vi "init.vi"(8 "error in (no error)":errorcluster, 11 "ILC_TC in":refnum<class "ILC_TC.lvclass">) -> (0 "error out":errorcluster, 3 "ILC_TC out":refnum<class "ILC_TC.lvclass">)   [LabVIEW 2013, in "ILC_TC.lvclass"]
uses:
  ILC_TC.lvclass
  <userlib>/Common/ILC/Configuration/ILC Serial.ctl
  <userlib>/Common/SerialProtocols/Configuration/SerialConfig.ctl
  <userlib>/Common/SerialProtocols/Configuration/SerialProtocol.ctl
  <userlib>/Common/SerialProtocols/Configuration/ProtocolParameters.ctl
  <userlib>/Common/SerialProtocols/Configuration/SerialMessageParameters.ctl
  <userlib>/Common/ILC/Configuration/ILC ADC.ctl
  <userlib>/Common/ILC/Configuration/InputChannels.ctl
  <userlib>/Common/ILC/Configuration/ScanRate_Hz_MultichannelOptions.ctl
  <userlib>/Common/ILC/ILC/ILC.lvclass/ILC.ctl
  <userlib>/Common/ILC/ILC/ILC.lvclass
  <userlib>/Common/SerialProtocols/SerialProtocols.lvlib
  <userlib>/Common/ILC/Configuration/ILCConfiguration.lvlib
  ConfigurationThisComponent/ConfigurationThisComponent.lvclass
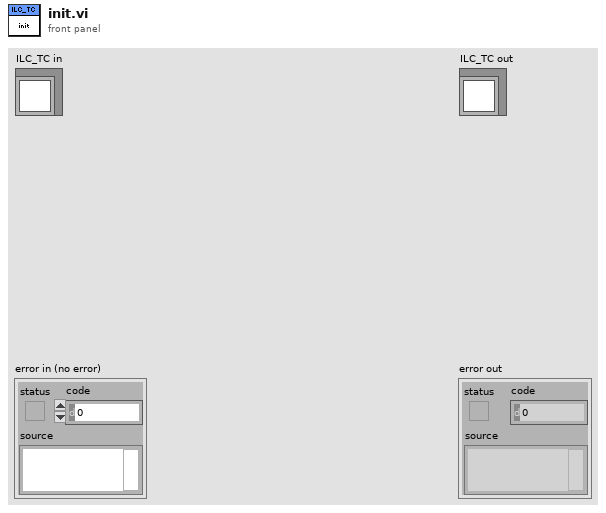
[diagram p1: front panel]
types:
  T1 = typedef "ILCCommon.lvlib/ILCConfiguration.lvlib/ILC ADC.ctl" = cluster{"Input Channels":T2, "Scan Rate (Hz) ":T3, "PGA Gain Coefficient":u8, "Reference Voltage Vref":dbl[unit], "Nominal Input Range in Counts":u32, "Preamplifier Gain":u8}
  T2 = typedef "ILCCommon.lvlib/ILCConfiguration.lvlib/InputChannels.ctl" = enum16{"Channel 0", "3 Channels", "5 Channels"}
  T3 = typedef "ILCCommon.lvlib/ILCConfiguration.lvlib/ScanRate_Hz_MultichannelOptions.ctl" = enum16{"50", "60", "100", "120", "200", "240", "300", "400", "480", "600", "1200", "2400", "4800"}
  T4 = typedef "ILCCommon.lvlib/ILCConfiguration.lvlib/ILC Serial.ctl" = cluster{"Serial":T5}
  T5 = typedef "SerialProtocols.lvlib/SerialConfig.ctl" = cluster{"Serial Protocol":T6, "Protocol Parameters":T7, "Serial Message Parameters":T8}
  T6 = typedef "SerialProtocols.lvlib/SerialProtocol.ctl" = enum16{"RS232", "RS485", "SerialSimulator"}
  T7 = typedef "SerialProtocols.lvlib/ProtocolParameters.ctl" = cluster{"VISA resource name":refnum<visa-resource-name>, "Baud Rate":u32, "Data Bits":u16, "Parity":enum16{"None", "Odd", "Even", "Mark", "Space"}, "Flow Control":u16, "Stop Bits":u16, "Timeout (ms)":u32}
  T8 = typedef "SerialProtocols.lvlib/SerialMessageParameters.ctl" = cluster{"Byte Count":u32, "Enable Termination Character":bool, "Termination Char":u8}
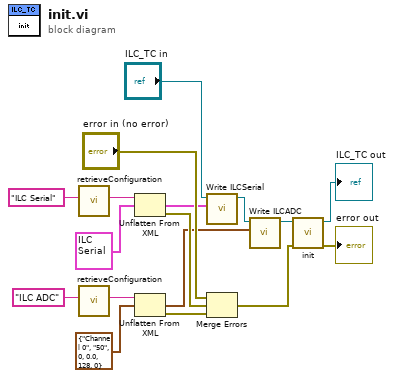
[diagram p0: block diagram]
diagram:
  n1 = call "retrieveConfiguration.vi"("configName"="ILC Serial") -> ("xmlConfig"=w12:string)  [unwired: 8 in, 2 out]
  n2 = call "retrieveConfiguration.vi"("configName"="ILC ADC") -> ("xmlConfig"=w10:string)  [unwired: 8 in, 2 out]
  n3 = Unflatten From XML(xml string=w12, type=T4 {"Serial"={"Serial Protocol"=enum."RS232", "Protocol Parameters"={"VISA resource name"="", "Baud Rate"=0, "Data Bits"=0, "Parity"=enum."None", "Flow Control"=0, "Stop Bits"=0, "Timeout (ms)"=0}, "Serial Message Parameters"={"Byte Count"=0, "Enable Termination Character"=FALSE, "Termination Char"=0}}} ("ILC")) -> (value=w3:T4, error out=w15:errorcluster)  [unwired: 1 in]
  n4 = Unflatten From XML(xml string=w10, type=T1 {"Input Channels"=enum."Channel 0", "Scan Rate (Hz) "=enum."50", "PGA Gain Coefficient"=0, "Reference Voltage Vref"=0.0, "Nominal Input Range in Counts"=128, "Preamplifier Gain"=0} ("ILC ADC")) -> (value=w2:T1, error out=w8:errorcluster)  [unwired: 1 in]
  n5 = call <userlib>:"Write ILCSerial.vi"("ILC Serial"=w3, "ILC in"="ILC_TC in") -> ("ILC out"=w5:refnum<class "ILC_TC.lvclass">)  [unwired: 9 in]
  n6 = Merge Errors("error in (no error)", w15, w8) -> (w1:errorcluster)
  n7 = call <userlib>:"Write ILCADC.vi"("ILC ADC"=w2, "ILC in"=w5) -> ("ILC out"=w4:refnum<class "ILC_TC.lvclass">)  [unwired: 9 in]
  n8 = call-parent "init.vi"("error in (no error)"=w1, "ILC in"=w4) -> ("error out"=→"error out":errorcluster, "ILC out"=→"ILC_TC out":refnum<class "ILC_TC.lvclass">)  [unwired: 8 in]
